vi "PSD.vi"(4 "error in (no error)":errorcluster caption="错误输入（无错误）", 6 "输入波形":waveform(dbl) caption="输出波形", 7 "dt":dbl) -> (0 "error out":errorcluster caption="错误输出", 1 "波形图":waveform(dbl)(graph)={"t0"=timestamp(0 s since 1904-01-01), "dt"=390.62499999999994, "Y"=[0.024471282958984375, 0.039576801615885296, 0.04980077593767322, 0.07337219982550662, 0.1424926016157528, 1.3754640529492843, 0.19434264234527268, 0.09398999193405373, 0.0632902391033216, 0.04831927291081195, 0.03938875539626057, 0.03337010934986245, 0.029124623425692362, 0.025872864670262015, 0.023331443482501768, 0.021279269350711588, 0.01961258181556757, 0.018170175529941355, 0.016979766456302923, 0.01592115465597211, 0.014984805311418844, 0.014183865729115435, 0.013472311035607892, 0.01284543243634929, 0.01223442163727234, 0.01173440221962791, 0.011177589286937892, 0.010771220769557452, 0.0103715989050219, 0.01000166229184351, 0.009650392462188448, 0.009335001478098182, 0.009039938355342643, 0.008766722931722351, 0.008499276487207564, 0.008257599315399758, 0.008029960396705263, 0.00787719975806492, 0.007624682401792018, 0.007467234576106422, 0.007279678355744929, 0.007104197988448805, 0.006906069815572803, 0.006783686454836766, 0.0066239458263320965, 0.006527160493892424, 0.006374064061419823, 0.006195440069801259, 0.0061388619476094655, 0.005981446528921198, 0.005886468484987766, 0.005802185891171443, 0.005693349086799617, 0.0056081395316140295, 0.005488028377302177, 0.005417172329491218, 0.0053291177442244516, 0.005253460029350709, 0.00517702697773943, 0.005110797518730482, 0.005056936995426669, 0.004983411794762686, 0.004930363769523166, 0.004868115718528812, 0.004799662347314822, 0.004716855815357289, 0.0046793174914304654, 0.004627252941896581, 0.004541689075502773, 0.004497892059274063, 0.004440583715342986, 0.00439126585466581, 0.004369327337929167, 0.004310200258407257, 0.004284326221824349, 0.00423892775040243, 0.00418862966356386, 0.00416289577367478, 0.004128638409110107, 0.0040956358224749105, 0.0040516763262554885, 0.0040242660595797165, 0.00398768900159714, 0.003963147353072002, 0.00393963956681302, 0.003917195400750559, 0.003860158869761374, 0.003833633154682015, 0.0038205083454820703, 0.003814258550211866, 0.003762553508196774, 0.003739648728299181, 0.003720326412396511, 0.0036632853844981946, 0.003643202653033845, 0.003656885275367599, 0.003645389854899682, 0.003623442361561301, 0.003604024955115401, 0.003584968182728699, 0.0035687476653787267, 0.0035552661304941563, 0.003548370825037908, 0.0035341034241564615, 0.0034971319104367344, 0.003510205575363794, 0.003456681986180992, 0.0034291327747217916, 0.003452531796324354, 0.0034346312726136912, 0.003426534698851254, 0.003436325582798964, 0.003458769413172076, 0.0034464781745900054, 0.0034104886971700983, 0.003410127065652215, 0.003407198464457342, 0.003393954186629053, 0.0033955627270477223, 0.00336512627935848, 0.0033797658050242372, 0.0033733281859413536, 0.0033531861629400588, 0.003392278393526379, 0.003358486206627685, 0.0033462625739087266, 0.003330167352482211, 0.0034688919748213846]})   [LabVIEW 2019]
uses:
  <vilib>/measure/maspectr.llb/FFT Spectrum (Real-Im) for 1 Chan.vi
  <vilib>/measure/NI_MAPro.lvlib
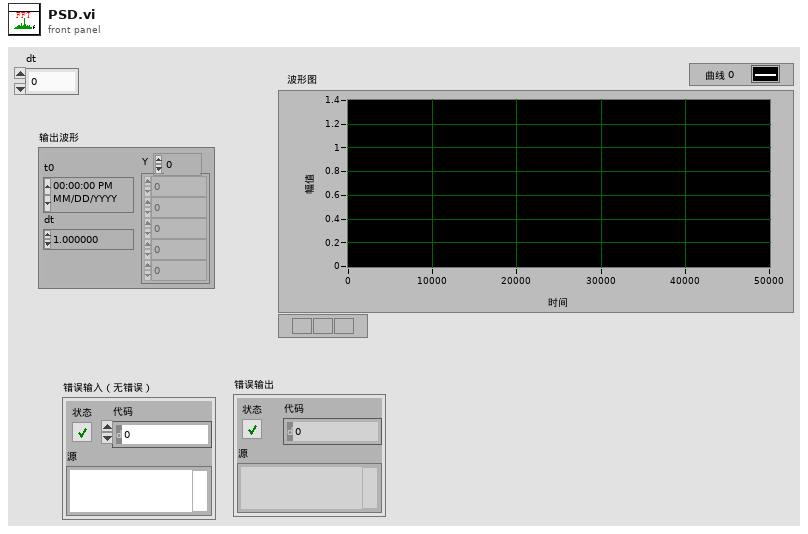
[diagram p1: front panel]
types:
  T1 = cluster{"f0":dbl, "df":dbl, "imaginary part":dbl[]}
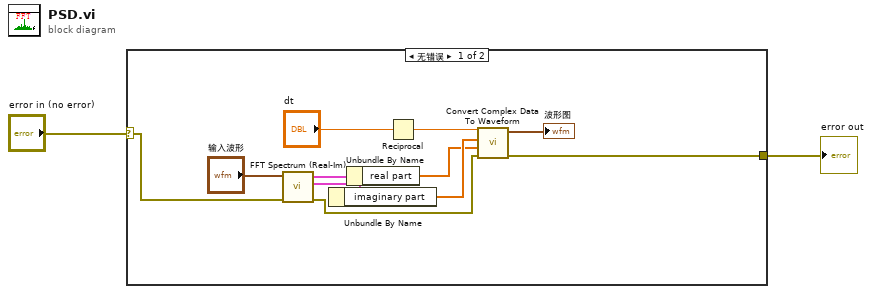
[diagram p0: block diagram]
diagram:
  n1 = case shown="无错误" "error in (no error)" {
    selector: "error in (no error)" -> [w5 w14]
    tunnel: [w3 w14] -> w1
    frame No Error {
      n2 = call-poly <vilib>:"FFT Spectrum (Real-Im).vi"("error in (no error)"=w5, "time signal"="输入波形") -> ("error out"=w4:errorcluster, "imaginary part"=w8:T1, "real part"=w9:cluster{"f0":dbl, "df":dbl, "real part":dbl[]})  [unwired: 5 in, 2 out]
      n3 = Unbundle By Name(w8) -> ("imaginary part"=w7:dbl[])
      n4 = Unbundle By Name(w9) -> ("real part"=w6:dbl[])
      n5 = Reciprocal(x="dt") -> (1/x=w12:dbl)
      n6 = call "Convert Complex Data To Waveform.vi"("error in"=w4, "Real Data"=w6, "Imaginary Data"=w7, "Sample Rate (S/s)"=w12) -> ("error out"=w3:errorcluster, "Waveform"=→"波形图":waveform(dbl))  [unwired: 6 in]
    }
    frame Error {
    }
  }
  "error out" <- w1
